vi "CRYAPI FILE.vi"(8 "sData":string="REGISTER", 9 "nData":i32, 10 "pVIRef":refnum<vi>, 11 "sAction":string="Basic") -> (0 "nData_Out":i32, 1 "sData_Out":string="REGISTER")   [LabVIEW 2013]
uses:
  CRYMain Sub Window Global.vi
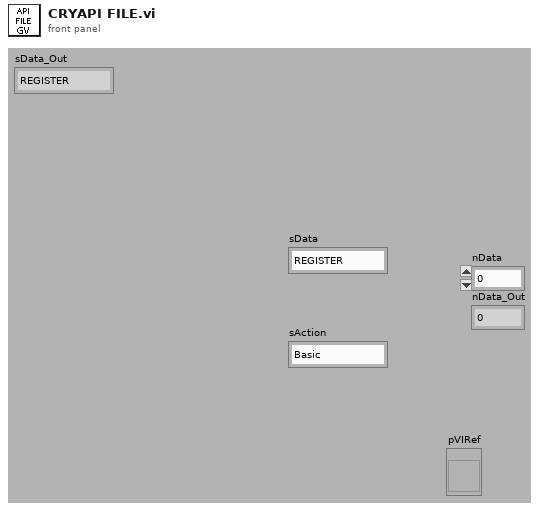
[diagram p1: front panel]
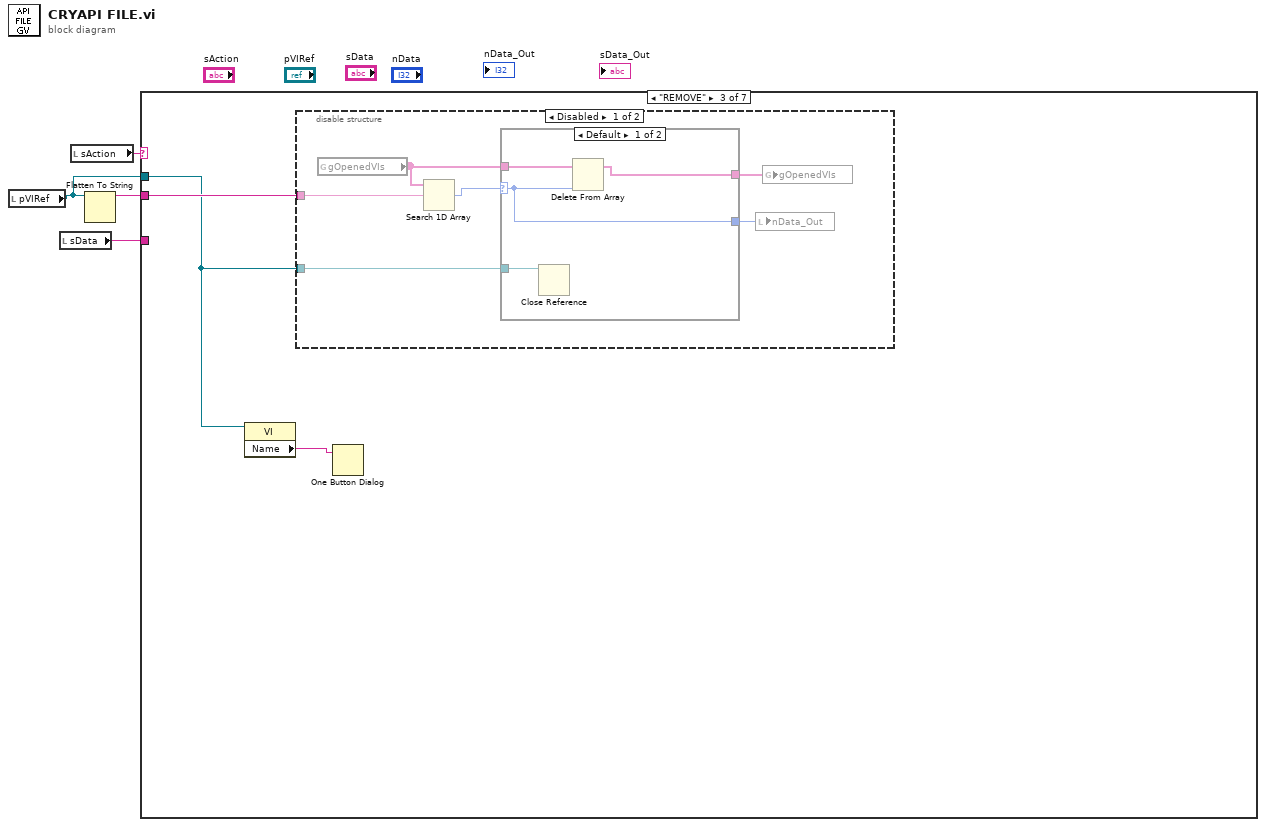
[diagram p0: block diagram]
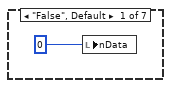
[diagram p2: hidden frame]
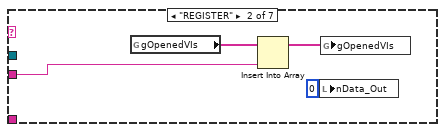
[diagram p3: hidden frame]
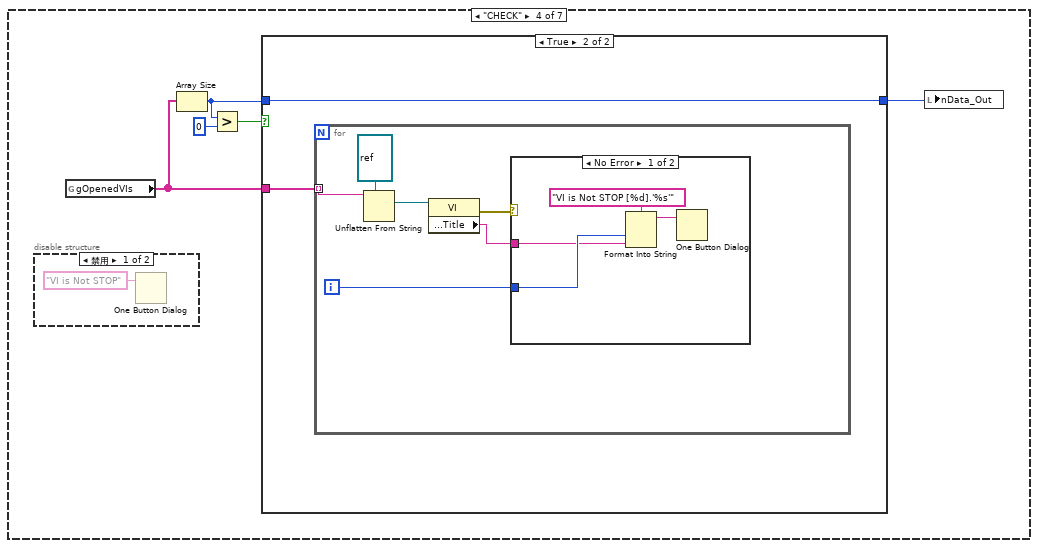
[diagram p6: hidden frame]
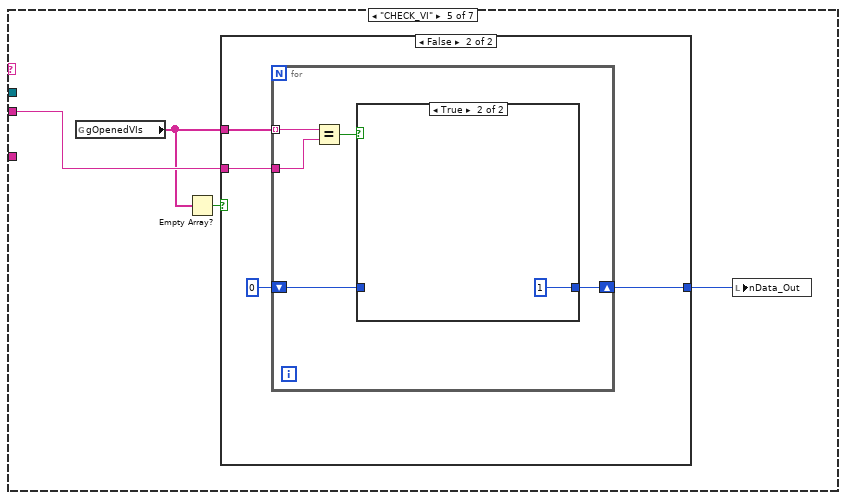
[diagram p10: hidden frame]
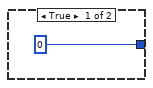
[diagram p11: hidden frame]
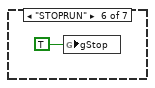
[diagram p13: hidden frame]
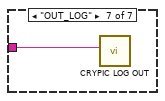
[diagram p14: hidden frame]
diagram:
  n1 = local read "pVIRef"() -> (w1:refnum<vi>)
  n2 = local read "sData"() -> (w3:string)
  n3 = local read "sAction"() -> (w4:string)
  n4 = Flatten To String(anything=w1) -> (data string=w2:string)  [unwired: 1 in, 4 out]
  n5 = case shown="\"REMOVE\"" w4 {
    tunnel: w3 -> [_ _ _ _ _ _ w61]
    tunnel: w2 -> [_ w6 w12 _ w47 _ _]
    tunnel: w1 -> [_ _ w11 _ _ _ _]
    frame "False", Default {
      n6 = local write "nData"(0 ("nData")) -> ()
    }
    frame "REGISTER" {
      n7 = global read "CRYMain Sub Window Global.vi" "gOpenedVIs"() -> (w9:string[])
      n8 = Insert Into Array(array=w9, new element=w6) -> (w8:string[])  [unwired: 1 in]
      n9 = local write "nData_Out"(0 ("nData_Out")) -> ()
      n10 = global write "CRYMain Sub Window Global.vi" "gOpenedVIs"(w8) -> ()
    }
    frame "REMOVE" {
      n11 = property class="VI"(reference=w11) -> ("Name"=w10:string)  [unwired: 1 in, 2 out]
      n12 = disable-structure shown="Disabled" {
        disable-tunnel: w12 -> [w15 _]
        disable-tunnel: w11 -> [w13 _]
        frame Disabled {
          n13 = global read "CRYMain Sub Window Global.vi" "gOpenedVIs"() -> (w17:string[])
          n14 = Search 1D Array(1D array=w17, element=w15) -> (index of element=w16:i32)  [unwired: 1 out]
          n15 = case shown="Default" w16 {
            selector: w16 -> [w21 w24]
            tunnel: w17 -> [w22 w23]
            tunnel: [w21 w24] -> w18
            tunnel: [w20 w23] -> w14
            tunnel: w13 -> [w19 _]
            frame Default {
              n16 = Close Reference(reference=w19) -> ()  [unwired: 1 in, 1 out]
              n17 = Delete From Array(array=w22, index=w21) -> (array with subset deleted=w20:string[])  [unwired: 1 in, 1 out]
            }
            frame -1 {
            }
          }
          n18 = local write "nData_Out"(w18) -> ()
          n19 = global write "CRYMain Sub Window Global.vi" "gOpenedVIs"(w14) -> ()
        }
        frame Enabled {
        }
      }
      n20 = One Button Dialog(message=w10) -> ()  [unwired: 1 in, 1 out]
    }
    frame "CHECK" {
      n21 = disable-structure shown="禁用" {
        frame Disabled {
          n22 = One Button Dialog(message="VI is Not STOP" ("initial string")) -> ()  [unwired: 2 out]
        }
        frame Enabled {
        }
      }
      n23 = global read "CRYMain Sub Window Global.vi" "gOpenedVIs"() -> (w25:string[])
      n24 = Array Size(array=w25) -> (size(s)=w27:i32)
      n25 = Greater?(x=w27, y=0) -> (0:w28:bool)
      n26 = case shown="True" w28 {
        tunnel: w25 -> [_ w33]
        tunnel: w27 -> [w31 w32]
        tunnel: [w31 w32] -> w26
        frame False {
        }
        frame True {
          n27 = for {
            tunnel: w33 -> [w37] mode=indexing
            i -> [w38]
            n28 = Unflatten From String(type=refnum<vi> refnum ("pVIRef"), binary string=w37) -> (value=w36:refnum<vi>)  [unwired: 1 in, 4 out]
            n29 = property class="VI"(reference=w36) -> (error out=w34:errorcluster, "Front Panel.Title"=w35:string)  [unwired: 1 in, 1 out]
            n30 = case shown="No Error" w34 {
              tunnel: w38 -> [w42 _]
              tunnel: w35 -> [w40 _]
              frame No Error {
                n31 = Format Into String(format string="VI is Not STOP [%d].'%s'", w42, w40) -> (resulting string=w41:string)  [unwired: 2 in, 1 out]
                n32 = One Button Dialog(message=w41) -> ()  [unwired: 2 out]
              }
              frame Error {
              }
            }
          }
        }
      }
      n33 = local write "nData_Out"(w26) -> ()
    }
    frame "CHECK_VI" {
      n34 = global read "CRYMain Sub Window Global.vi" "gOpenedVIs"() -> (w45:string[])
      n35 = Empty Array?(array=w45) -> (empty?=w46:bool)
      n36 = case shown="False" w46 {
        tunnel: w45 -> [_ w52]
        tunnel: w47 -> [_ w50]
        tunnel: [0 ("nData_Out") w49] -> w44
        frame True {
        }
        frame False {
          n37 = for {
            tunnel: w52 -> [w57] mode=indexing
            shift-right: [w55] -> w49
            shift-left: 0 ("nData_Out") -> [w56]
            tunnel: w50 -> [w53]
            n38 = Equal?(x=w57, y=w53) -> (x = y?=w54:bool)
            n39 = case shown="True" w54 {
              tunnel: w56 -> [w58 _]
              tunnel: [w58 1 ("nData_Out")] -> w55
              frame False {
              }
              frame True {
              }
            }
          }
        }
      }
      n40 = local write "nData_Out"(w44) -> ()
    }
    frame "STOPRUN" {
      n41 = global write "CRYMain Sub Window Global.vi" "gStop"(TRUE ("gStop")) -> ()
    }
    frame "OUT_LOG" {
      n42 = call "CRYPIC LOG OUT.vi"("sData"=w61) -> ()  [unwired: 11 in]
    }
  }
